vi "Queue Example.vi"() -> ()   [LabVIEW 2017]
panel:
  out "error out":errorcluster
  out "element":dbl
  in  "stop":bool
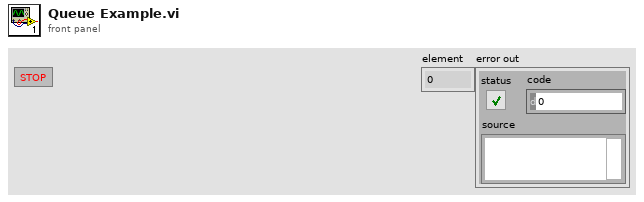
[diagram p1: front panel]
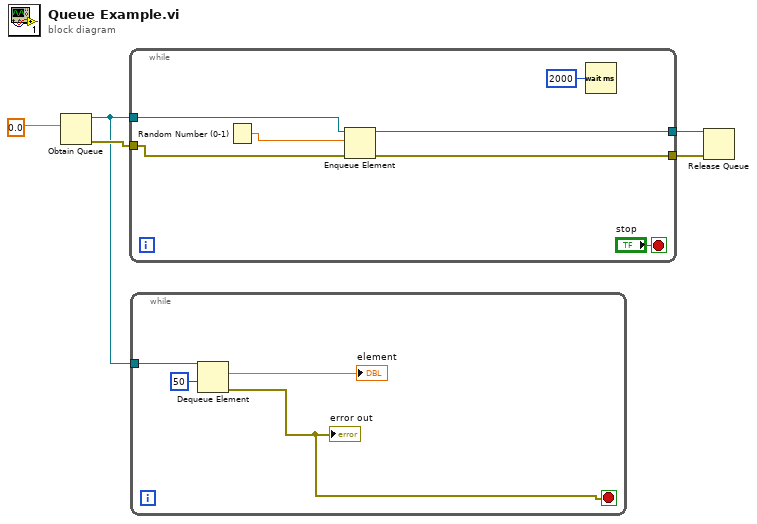
[diagram p0: block diagram]
diagram:
  n1 = Obtain Queue(element data type=0.0 ("number (0 to 1)")) -> (queue out=w1:refnum<queue>, error out=w5:errorcluster)  [unwired: 4 in, 1 out]
  n2 = while {
    tunnel: w1 -> [w10]
    tunnel: w5 -> [w9]
    tunnel: [w8] -> w2
    tunnel: [w7] -> w3
    stop <- "stop" stop-if-true
    n3 = Random Number (0-1)() -> (number: 0 to 1=w11:dbl)
    n4 = Enqueue Element(queue=w10, element=w11, error in (no error)=w9) -> (queue out=w8:refnum<queue>, error out=w7:errorcluster)  [unwired: 1 in, 1 out]
    n5 = Wait (ms)(milliseconds to wait=u32 2000) -> ()  [unwired: 1 out]
  }
  n6 = while {
    tunnel: w1 -> [w16]
    stop <- w13 stop-if-true
    n7 = Dequeue Element(queue=w16, timeout in ms (-1)=50) -> (element=→"element":dbl, error out=w13:errorcluster)  [unwired: 1 in, 2 out]
    "error out" <- w13
  }
  n8 = Release Queue(queue=w2, error in (no error)=w3) -> ()  [unwired: 1 in, 3 out]
